vi "Set configuration chain.vi"(8 "error in (no error)":errorcluster, 9 "class names":string[](array[string]), 10 "configuration":variant[](array[variant]), 11 "Thorcam in":refnum<class "Thorcam.lvclass">) -> (0 "error out":errorcluster, 3 "Thorcam out":refnum<class "Thorcam.lvclass">)   [LabVIEW 2012, in "Thorcam.lvclass"]
uses:
  Thorcam.lvclass
  <vilib>/Distrio/Murmex/Murmex/Murmex.lvclass
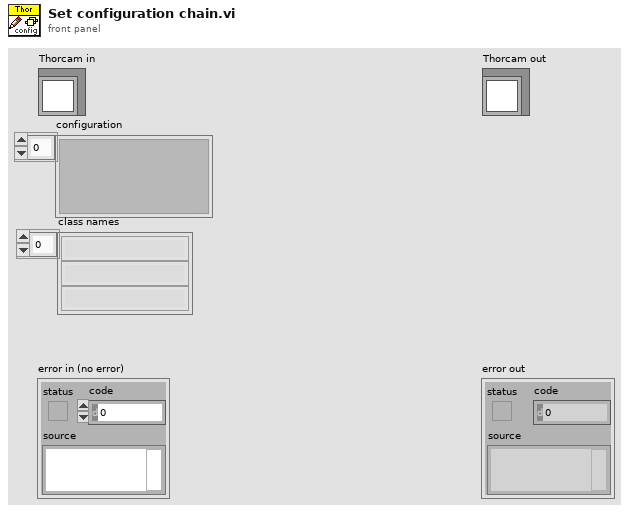
[diagram p1: front panel]
types:
  T1 = typedef "Thorcam.lvclass/configuration.ctl" = cluster{"camera ID1":u32, "Settings":string, "Cross Correlation method":T2, "Reporting folder":path, "LUT":path, "Stage component":string, "Background image":path, "camera ID2":u32, "select camera":u32, "Shift to defocus conversion factor":dbl, "Alignment quality threshold":dbl}
  T2 = typedef "Thorcam.lvclass/cross correlation method.ctl" = enum16{"default", "normalised cross correlation", "normalised mutual information", "binary cross correlation", "binary mutual information"}
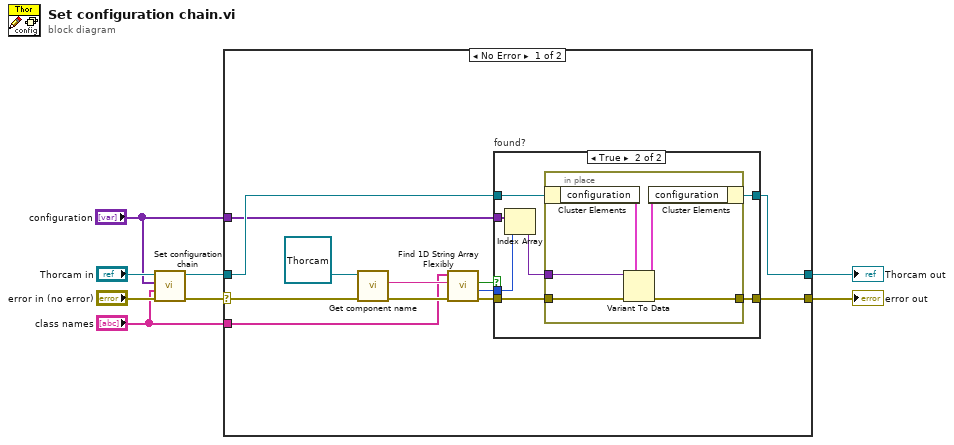
[diagram p0: block diagram]
diagram:
  n1 = call-parent "Set configuration chain.vi"("error in (no error)"="error in (no error)", "class names"="class names", "configuration"="configuration", "Murmex in"="Thorcam in") -> ("error out"=w6:errorcluster, "Murmex out"=w3:refnum<class "Thorcam.lvclass">)  [unwired: 6 in]
  n2 = case shown="No Error" w6 {
    selector: w6 -> [w14 w36]
    tunnel: [w15 w36] -> w5
    tunnel: [w9 w35] -> w4
    tunnel: w3 -> [w12 w35]
    tunnel: "class names" -> [w13 _]
    tunnel: "configuration" -> [w11 _]
    frame No Error {
      n3 = call <vilib>:"Get component name.vi"("error in (no error)"=w14, "Murmex in"=refnum<class "Thorcam.lvclass"> refnum ("Thorcam in")) -> ("error out"=w20:errorcluster, "component name"=w18:string)  [unwired: 7 in, 1 out]
      n4 = call <vilib>:"Find 1D String Array Flexibly.vi"("error in (no error)"=w20, "element"=w18, "array"=w13) -> ("error out"=w19:errorcluster, "index of element"=w17:i32, "found?"=w16:bool)  [unwired: 6 in]
      n5 = case "found?" shown="True" w16 {
        tunnel: w11 -> [_ w29]
        tunnel: w12 -> [w22 w27]
        tunnel: [w22 w26] -> w9
        tunnel: [w21 w25] -> w15
        tunnel: w19 -> [w21 w24]
        tunnel: w17 -> [_ w23]
        frame False {
        }
        frame True {
          n6 = Index Array(array=w29, index=w23) -> (element=w28:variant)
          n7 = in-place {
            in-place-border: w28 -> [w34]
            in-place-border: w24 -> [w32]
            in-place-border: [w30] -> w25
            n8 = in-place-cluster #1(w27) -> ("configuration"=w33:T1)
            n9 = Variant To Data(error in=w32, type=w33, Variant=w34) -> (data=w31:T1, error out=w30:errorcluster)
            n10 = in-place-cluster #1("configuration"=w31) -> (w26:refnum<class "Thorcam.lvclass">)
          }
        }
      }
    }
    frame Error {
    }
  }
  "error out" <- w5
  "Thorcam out" <- w4
